vi "PAN_CreateDir.vi"(7 "error in":errorcluster, 10 "dir to create":path) -> (0 "error":errorcluster, 3 "dir  out":path)   [LabVIEW 2016]
doc: "This VI will examine the directory given and will create it if it does not exists."
panel:
  in  "sep":string="/"
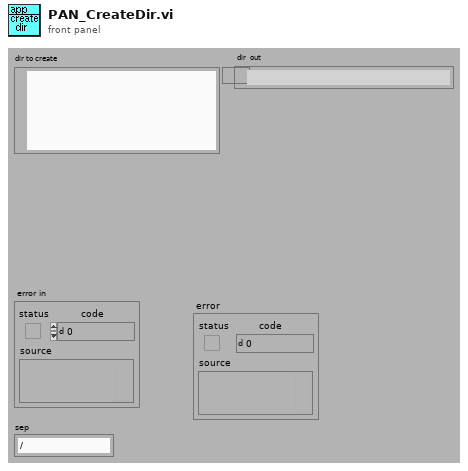
[diagram p1: front panel]
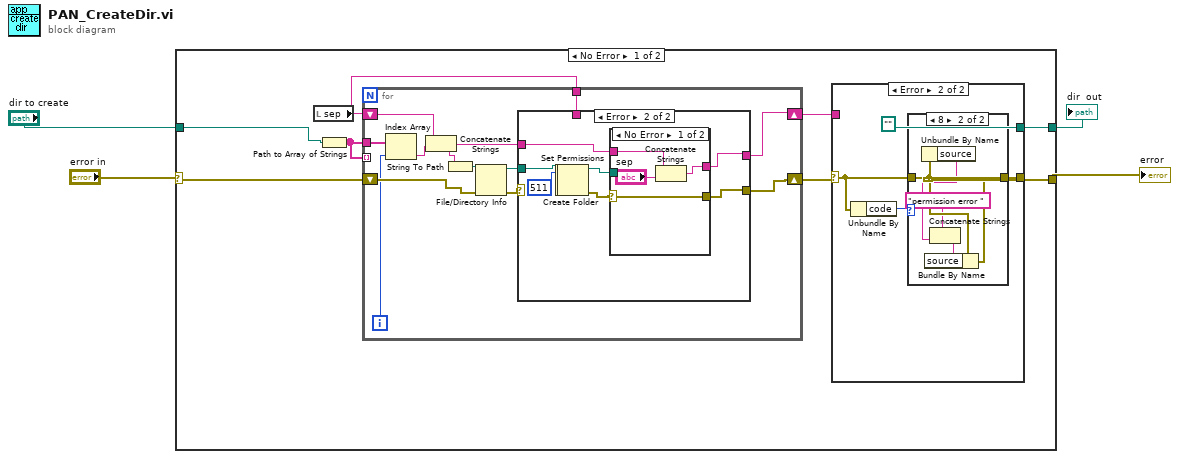
[diagram p0: block diagram]
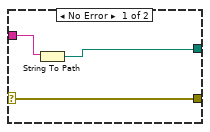
[diagram p2: hidden frame]
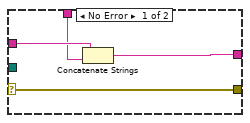
[diagram p4: hidden frame]
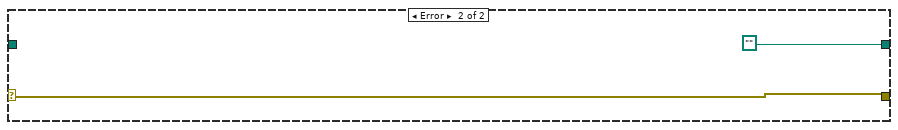
[diagram p6: hidden frame]
diagram:
  n1 = case shown="No Error" "error in" {
    selector: "error in" -> [w6 w58]
    tunnel: [w11 path ""] -> w4
    tunnel: "dir to create" -> [w5 _]
    tunnel: [w10 w58] -> w3
    frame No Error {
      n2 = local read "sep"() -> (w7:string)
      n3 = Path to Array of Strings(0:w5) -> (2:w9:string[])  [unwired: 1 out]
      n4 = for {
        shift-right: [w33] -> w12
        shift-left: w6 -> [w34]
        shift-right: [w28] -> w8
        shift-left: w7 -> [w29]
        tunnel: w9 -> [w27]
        tunnel: w9 -> [_] mode=indexing
        tunnel: w7 -> [w26]
        i -> [w32]
        n5 = Index Array(array=w27, index=w32) -> (element=w30:string)
        n6 = Concatenate Strings(w29, w30) -> (w31:string)
        n7 = String To Path(string=w31) -> (path=w37:path)
        n8 = File/Directory Info(path=w37, error in=w34) -> (path out=w35:path, error out=w36:errorcluster)  [unwired: 5 out]
        n9 = case shown="Error" w36 {
          selector: w36 -> [w41 _]
          tunnel: [w39 w48] -> w28
          tunnel: w35 -> [_ w50]
          tunnel: [w41 w47] -> w33
          tunnel: w31 -> [w40 w46]
          tunnel: w26 -> [w38 _]
          frame No Error {
            n10 = Concatenate Strings(w40, w38) -> (w39:string)
          }
          frame Error {
            n11 = Create Folder(path (use dialog)=w50) -> (created path=w43:path, error out=w42:errorcluster)  [unwired: 1 in, 2 out]
            n12 = Set Permissions(7:i16 511 ("permissions"), 8:w42, 11:w43) -> (0:w49:errorcluster, 3:w45:path)  [unwired: 2 out]
            n13 = case shown="No Error" w49 {
              selector: w49 -> [w54 w56]
              tunnel: [w52 w55] -> w48
              tunnel: [w54 w56] -> w47
              tunnel: w46 -> [w53 w55]
              tunnel: w45 -> [_ _]
              frame No Error {
                n14 = Concatenate Strings(w53, "sep") -> (w52:string)
              }
              frame Error {
              }
            }
          }
        }
      }
      n15 = case shown="Error" w12 {
        selector: w12 -> [w15 w17]
        tunnel: [w13 path ""] -> w11
        tunnel: [w15 w16] -> w10
        tunnel: w8 -> [w14 _]
        frame No Error {
          n16 = String To Path(string=w14) -> (path=w13:path)
        }
        frame Error {
          n17 = Unbundle By Name(w17) -> ("code"=w18:i32)
          n18 = case shown="8" w18 {
            tunnel: w17 -> [w20 w25]
            tunnel: [w20 w24] -> w16
            frame Default {
            }
            frame 8 {
              n19 = Unbundle By Name(w25) -> ("source"=w22:string)
              n20 = Concatenate Strings("permission error " ("string"), w22) -> (w21:string)
              n21 = Bundle By Name(cluster=w25, "source"=w21) -> (w24:errorcluster)
            }
          }
        }
      }
    }
    frame Error {
    }
  }
  "dir  out" <- w4
  "error" <- w3
